vi "SPD.HV_Grid Min Search.vi"(7 "Continue":refnum<vi>, 8 "Error In":errorcluster, 9 "min step":dbl=32.0 format="%#_13g", 10 "HV_GridParams":T1, 11 "SPD.Stand Ctrl in":T2 {"spdDeviceSession"."hidSPD.Sturtup Values"."HV_bias" format="%#_6p, V"; "spdDeviceSession"."hidSPD.Sturtup Values"."TSet" format="%#_6p, DegC"; "spdDeviceSession"."hidSPD.Controller"."HV_bias" format="%#_6p, V"; "spdDeviceSession"."hidSPD.Controller"."TSet" format="%#_6p, DegC"}) -> (0 "Error Out":errorcluster, 1 "pass":bool, 2 "HV_bias min":dbl, 3 "SPD.Stand Ctrl out":T2 {"spdDeviceSession"."hidSPD.Sturtup Values"."HV_bias" format="%#_6p, V"; "spdDeviceSession"."hidSPD.Sturtup Values"."TSet" format="%#_6p, DegC"; "spdDeviceSession"."hidSPD.Controller"."HV_bias" format="%#_6p, V"; "spdDeviceSession"."hidSPD.Controller"."TSet" format="%#_6p, DegC"})   [LabVIEW 2018]
uses:
  typedefs/SPD.Stand Ctrl.ctl
  Instruments/SPD HID Interface/hidSPDLibForLabView/LibVIs/hidSPD Controls/hidSPD Device Session.ctl
  Instruments/SPD HID Interface/hidSPDLibForLabView/LibVIs/hidSPD Controls/hidSPD Controller.ctl
  Instruments/SPD HID Interface/hidSPDLibForLabView/LibVIs/hidSPD Controls/hidSPD SPD Type.ctl
  Instruments/KC705 DevBoard/typedefs/DevB.Session.ctl
  Instruments/KeySight 53230A/typedefs/FreqC.Session.ctl
  Instruments/KeySight 8164B/KeySight 8164B LAN InstrLib/typedefs/KeySight 8164B control.ctl
  Instruments/LeCroy SDA830/typedefs/LeCroy.Session.ctl
  typedefs/SPD.Events.ctl
  ConfigFile/SPD.Config File ctrl.ctl
  <vilib>/Utility/config.llb/Config Data RefNum.ctl
  typedefs/SPD.Meas Result.ctl
  typedefs/SPD.Queues.ctl
  typedefs/SPD.Stand state.ctl
  typedefs/SPD.HV_Grid Test Params.ctl
  SubVIs/comparison mode.ctl
  SubVIs/Min_Max.ctl
  Instruments/KeySight 8164B/KeySight 8164B LAN InstrLib.lvlib
  <vilib>/Utility/config.llb/NI_LVConfig.lvlib
  Instruments/SPD HID Interface/hidSPDLibForLabView/hidSPDLibForLabView.lvlib
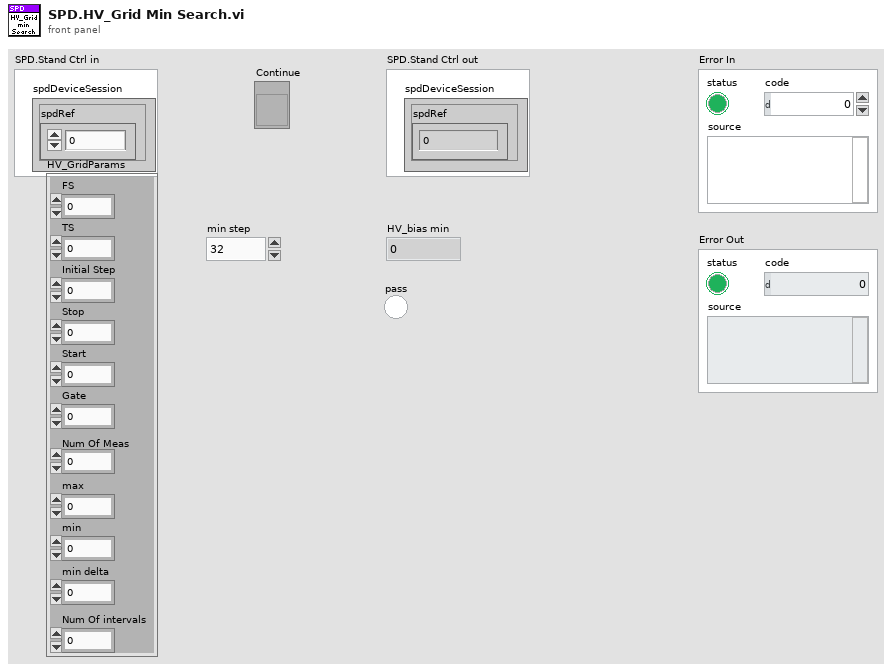
[diagram p1: front panel]
types:
  T1 = typedef "SPD.HV_Grid Test Params.ctl" = cluster{"FS":i32, "TS":i32, "Initial Step":dbl, "Stop":dbl, "Start":dbl, "Gate":dbl, "Num Of Meas":i32, "max":dbl, "min":dbl, "min delta":dbl, "Num Of intervals":i32}
  T2 = typedef "SPD.Stand Ctrl.ctl" = cluster{"spdDeviceSession":T3, "DevBSession":T6, "FreqCSession":T7, "8164BSession":T8, "LeCroySession":T9, "Events":T10, "configFile":T11, "SPD.Result":T13, "SPD.Queues":T14, "Console":refnum<vi>}
  T3 = typedef "hidSPDLibForLabView.lvlib/hidSPD Device Session.ctl" = cluster{"spdRef":u64, "connected":bool, "spdName":string, "hidSPD.Controller":T4, "hidSPD.Sturtup Values":T4, "SPD Type":T5}
  T4 = typedef "hidSPDLibForLabView.lvlib/hidSPD Controller.ctl" = cluster{"TSet":sgl, "HV_bias":sgl, "DDS_stb_code":u16}
  T5 = typedef "hidSPDLibForLabView.lvlib/hidSPD SPD Type.ctl" = enum16{"Free Run", "Gate"}
  T6 = typedef "DevB.Session.ctl" = cluster{"DevBRef":refnum<visa-resource-name>, "connected":bool}
  T7 = typedef "FreqC.Session.ctl" = cluster{"FreqCRef":refnum<visa-resource-name>, "timeout":dbl, "Gate":dbl, "connected":bool}
  T8 = typedef "KeySight 8164B LAN InstrLib.lvlib/KeySight 8164B control.ctl" = cluster{"Connection ID":refnum<k5>, "Connected":bool, "Info":string, "Slots Info":string[]}
  T9 = typedef "LeCroy.Session.ctl" = cluster{"LeCroySession":refnum<visa-resource-name>, "connected":bool}
  T10 = typedef "SPD.Events.ctl" = cluster{"DCRTest":refnum<user-event>, "Stop":refnum<user-event>}
  T11 = typedef "SPD.Config File ctrl.ctl" = cluster{"configFile ref":T12, "configFile path":path, "equipmentFile ref":T12}
  T12 = typedef "NI_LVConfig.lvlib/Config Data RefNum.ctl" = refnum<k1>
  T13 = typedef "SPD.Meas Result.ctl" = cluster{"HV_Bias":dbl[][][], "Stb_code":dbl[], "Temprature":dbl[], "Data":dbl[][][][], "DateTime":string}
  T14 = typedef "SPD.Queues.ctl" = cluster{"state queue":refnum<queue>}
  T15 = typedef "Min_Max.ctl" = cluster{"min":dbl, "max":dbl}
  T16 = typedef "comparison mode.ctl" = enum16{"in range", "bigger then min", "bigger then max", "less then min", "less then max"}
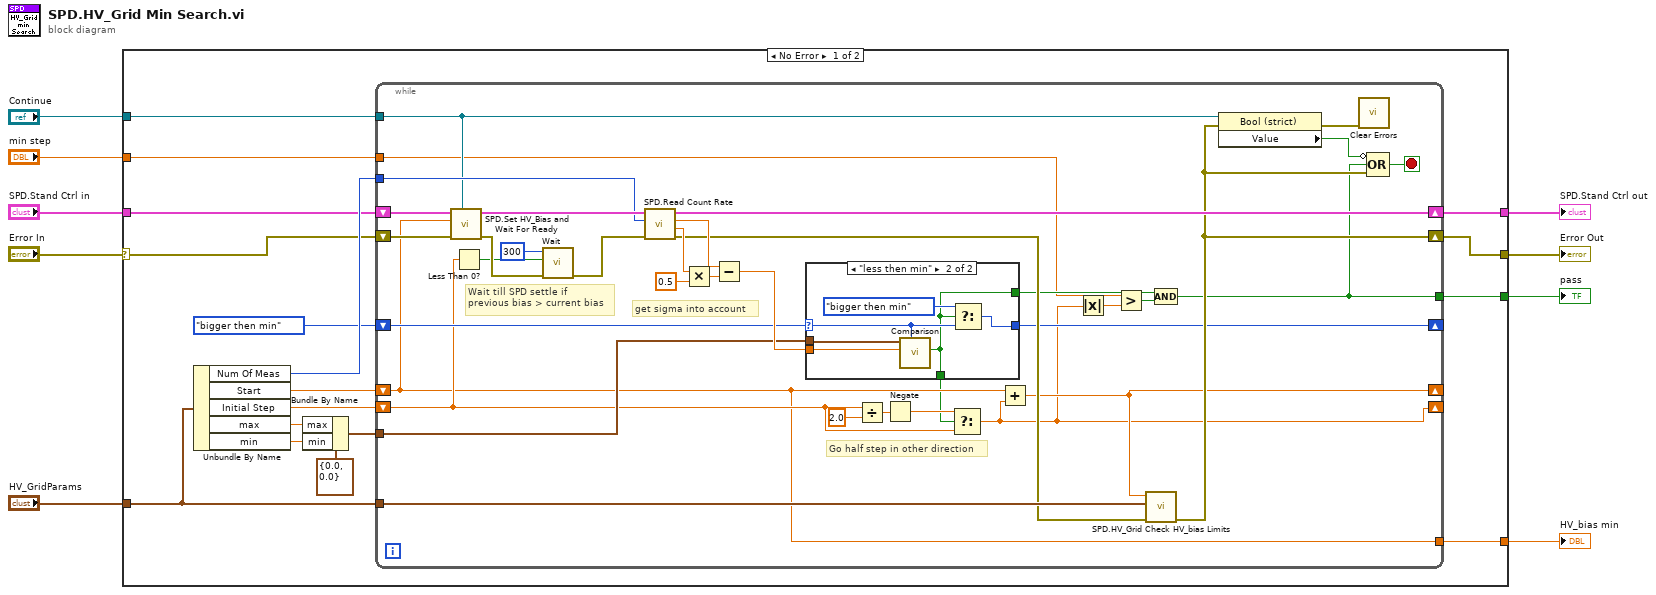
[diagram p0: block diagram]
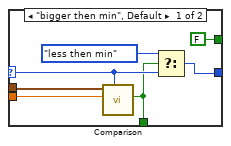
[diagram p2: hidden frame]
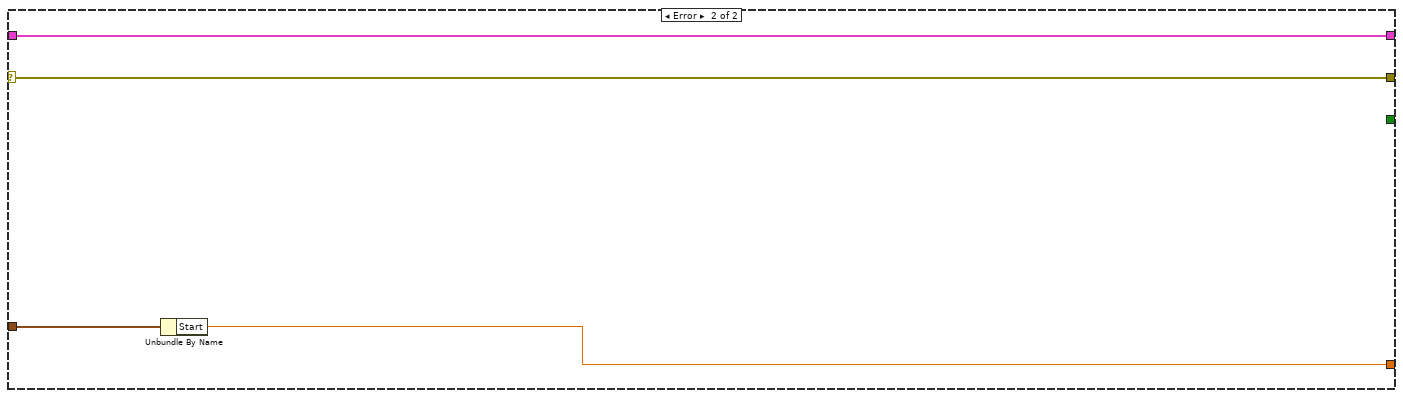
[diagram p3: hidden frame]
diagram:
  n1 = case shown="No Error" "Error In" {
    selector: "Error In" -> [w10 w79]
    tunnel: "Continue" -> [w26 _]
    tunnel: "SPD.Stand Ctrl in" -> [w23 w80]
    tunnel: [w22 w80] -> w7
    tunnel: [w21 w79] -> w6
    tunnel: "HV_GridParams" -> [w20 w78]
    tunnel: [w18 w77] -> w4
    tunnel: [w12 _] -> w3
    tunnel: "min step" -> [w11 _]
    frame No Error {
      n2 = Unbundle By Name(w20) -> ("Num Of Meas"=w25:i32, "Start"=w24:dbl, "Initial Step"=w13:dbl, "max"=w16:dbl, "min"=w15:dbl)
      n3 = Bundle By Name(cluster=T15 {"min"=0.0, "max"=0.0} ("minMax"), "max"=w16, "min"=w15) -> (w14:T15)
      n4 = while {
        tunnel: w26 -> [w51]
        tunnel: w25 -> [w62]
        shift-right: [w56] -> w22
        shift-left: w23 -> [w57]
        shift-right: [w33] -> _
        shift-left: w24 -> [w39]
        shift-right: [w50] -> w21
        shift-left: w10 -> [w55]
        tunnel: w20 -> [w54]
        shift-right: [w29] -> _
        shift-left: w13 -> [w41]
        shift-right: [w38] -> _
        shift-left: comparison_mode."bigger then min" ("Comparison Mode") -> [w43]
        tunnel: [w39] -> w18
        tunnel: w14 -> [w42]
        tunnel: w11 -> [w30]
        tunnel: [w28] -> w12
        stop <- w53 stop-if-true
        # "Go half step in other direction"
        # "get sigma into account"
        # "Wait till SPD settle if \nprevious bias > current bias"
        n5 = call "SPD.Set HV_Bias and Wait For Ready.vi"("Continue"=w51, "Error In"=w55, "HV_Bias"=w39, "SPD.Stand Ctrl in"=w57) -> ("Error Out"=w45:errorcluster, "SPD.Stand Ctrl out"=w63:T2)  [unwired: 6 in]
        n6 = Less Than 0?(x=w41) -> (x < 0?=w44:bool)
        n7 = call "Wait.vi"("error in (no error)"=w45, "wait? (true)"=w44, "milliseconds to wait"=u32 300) -> ("error out"=w47:errorcluster)  [unwired: 8 in]
        n8 = call "SPD.Read Count Rate.vi"("Error In"=w47, "Num of Meas"=w62, "SPD.Stand Ctrl in"=w63) -> ("Error Out"=w40:errorcluster, "Count sigma"=w59:dbl, "Count"=w58:dbl, "SPD.Stand Ctrl out"=w56:T2)  [unwired: 5 in]
        n9 = Multiply(x=w59, y=0.5) -> (x*y=w61:dbl)
        n10 = Subtract(x=w58, y=w61) -> (x-y=w52:dbl)
        n11 = case shown="\"less then min\"" w43 {
          selector: w43 -> [w68 w74]
          tunnel: w52 -> [w70 w76]
          tunnel: w42 -> [w69 w75]
          tunnel: [w66 w72] -> w38
          tunnel: [w65 w71] -> w35
          tunnel: [FALSE w71] -> w32
          frame "bigger then min", Default {
            n12 = call "Comparison.vi"("Comparison Mode"=w68, "value"=w70, "minMax"=w69) -> ("result"=w65:bool)  [unwired: 8 in]
            n13 = Select(t=comparison_mode."less then min", s=w65, f=w68) -> (s? t:f=w66:T16)
          }
          frame "less then min" {
            n14 = call "Comparison.vi"("Comparison Mode"=w74, "value"=w76, "minMax"=w75) -> ("result"=w71:bool)  [unwired: 8 in]
            n15 = Select(t=comparison_mode."bigger then min", s=w71, f=w74) -> (s? t:f=w72:T16)
          }
        }
        n16 = Divide(x=w41, y=2.0) -> (x/y=w36:dbl)
        n17 = Negate(x=w36) -> (-x=w37:dbl)
        n18 = Select(t=w37, s=w35, f=w41) -> (s? t:f=w29:dbl)
        n19 = Add(x=w39, y=w29) -> (x+y=w33:dbl)
        n20 = Absolute Value(x=w29) -> (abs(x)=w27:dbl)
        n21 = Greater?(x=w30, y=w27) -> (0:w31:bool)
        n22 = call "SPD.HV_Grid Check HV_bias Limits.vi"("Error In"=w40, "HV_GridParams"=w54, "Next HV_bias"=w33) -> ("Error Out"=w50:errorcluster)  [unwired: 8 in]
        n23 = Compound Arithmetic op=AND(w32, w31) -> (w28:bool)
        n24 = property class="Bool (strict)"(reference=w51, error in=w50) -> (error out=w48:errorcluster, "Value"=w49:bool)  [unwired: 1 out]
        n25 = call <vilib>:"Clear Errors.vi"("error in (no error)"=w48) -> ()  [unwired: 5 in, 2 out]
        n26 = Compound Arithmetic op=OR(invert w49, w28, w50) -> (w53:bool)
      }
    }
    frame Error {
      n27 = Unbundle By Name(w78) -> ("Start"=w77:dbl)
    }
  }
  "SPD.Stand Ctrl out" <- w7
  "Error Out" <- w6
  "HV_bias min" <- w4
  "pass" <- w3
